vi "UDP Discovery Server.vi"(0 "Name":string, 7 "Port":u16) -> (15 "error out":errorcluster)   [LabVIEW 2020]
uses:
  <vilib>/Utility/tcp.llb/UDP Multicast Read-Write Open.vi
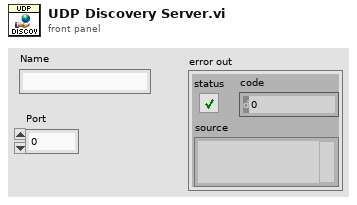
[diagram p1: front panel]
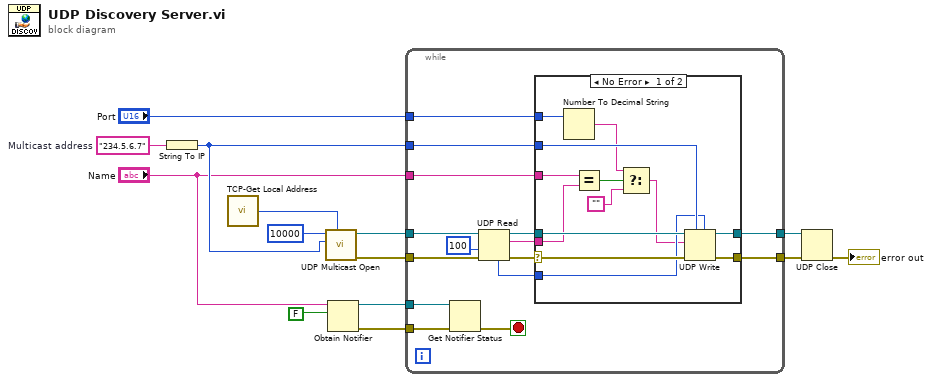
[diagram p0: block diagram]
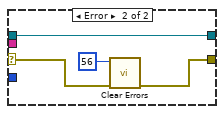
[diagram p2: hidden frame]
diagram:
  w10 = "234.5.6.7"  # Multicast address
  n1 = String To IP(1:w10) -> (0:w8:u32)
  n2 = call "TCP-Get Local Address.vi"() -> ("net address"=w1:u32)  [unwired: 14 in, 1 out]
  n3 = call-poly <vilib>:"UDP Multicast Open.vi"("net address"=w1, "multicast addr"=w8, "port"=u16 10000) -> ("error out"=w12:errorcluster, "connection ID"=w11:refnum<k16>)  [unwired: 6 in, 1 out]
  n4 = Obtain Notifier(name (unnamed)="Name", notification data type=FALSE) -> (notifier out=w3:refnum<notifier>, error out=w2:errorcluster)  [unwired: 2 in, 1 out]
  n5 = while {
    tunnel: w11 -> [w29]
    tunnel: w12 -> [w28]
    tunnel: [w27] -> w13
    tunnel: [w26] -> w14
    tunnel: "Name" -> [w25]
    tunnel: w8 -> [w24]
    tunnel: "Port" -> [w18]
    tunnel: w3 -> [w17]
    tunnel: w2 -> [w16]
    stop <- w15 stop-if-true
    n6 = Get Notifier Status(notifier=w17, error in (no error)=w16) -> (error out=w15:errorcluster)  [unwired: 4 out]
    n7 = UDP Read(connection ID=w29, timeout ms (25000)=100, 8:w28) -> (data out=w21:string, error out=w22:errorcluster, 3:w20:refnum<k16>, 4:w19:u16)  [unwired: 2 out]
    n8 = case shown="No Error" w22 {
      selector: w22 -> [w38 w46]
      tunnel: [w39 w44] -> w27
      tunnel: w21 -> [w36 _]
      tunnel: w25 -> [w42 _]
      tunnel: w20 -> [w41 w43]
      tunnel: [w40 w43] -> w26
      tunnel: w24 -> [w37 _]
      tunnel: w19 -> [w35 _]
      tunnel: w18 -> [w31 _]
      frame No Error {
        n9 = Number To Decimal String(number=w31) -> (decimal integer string=w30:string)  [unwired: 1 in]
        n10 = Equal?(x=w42, y=w36) -> (x = y?=w34:bool)
        n11 = Select(t=w30, s=w34, f="") -> (s? t:f=w32:string)
        n12 = UDP Write(address=w37, port or service name=w35, connection ID=w41, data in=w32, 8:w38) -> (error out=w39:errorcluster, 3:w40:refnum<k16>)  [unwired: 1 in]
      }
      frame Error {
        n13 = call <vilib>:"Clear Errors.vi"("error in (no error)"=w46, "specific error code to clear (0: all)"=56) -> ("error out"=w44:errorcluster)  [unwired: 4 in, 1 out]
      }
    }
  }
  n14 = UDP Close(connection ID=w14, 8:w13) -> (error out=→"error out":errorcluster)  [unwired: 1 out]
